vi "disableGrey.vi"(0 "Disable 1":refnum<vi>, 1 "Disable 2":refnum<vi>, 2 "Disable 3":refnum<vi>, 3 "error in (no error)":errorcluster, 4 "Enable this":refnum<vi>) -> (5 "error out":errorcluster)   [LabVIEW 2018]
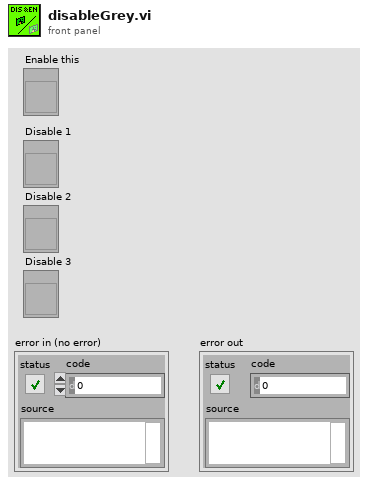
[diagram p1: front panel]
types:
  T1 = enum8{"Enabled", "Disabled", "Disabled and Grayed Out"}
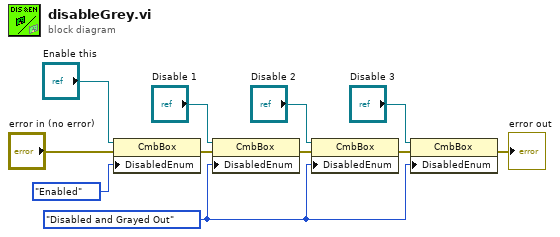
[diagram p0: block diagram]
diagram:
  w10 = T1."Disabled and Grayed Out" ("Disabled")
  n1 = property on="Property Node" class="CmbBox"(reference="Enable this", error in="error in (no error)", "DisabledEnum"=T1."Enabled" ("Disabled")) -> (error out=w7:errorcluster)  [unwired: 1 out]
  n2 = property on="Property Node" class="CmbBox"(reference="Disable 1", error in=w7, "DisabledEnum"=w10) -> (error out=w8:errorcluster)  [unwired: 1 out]
  n3 = property on="Property Node" class="CmbBox"(reference="Disable 2", error in=w8, "DisabledEnum"=w10) -> (error out=w9:errorcluster)  [unwired: 1 out]
  n4 = property on="Property Node" class="CmbBox"(reference="Disable 3", error in=w9, "DisabledEnum"=w10) -> (error out=→"error out":errorcluster)  [unwired: 1 out]
